vi "CreateNewMissions.vi"(4 "Timeout (s)":dbl, 6 "Duration (s)\n[For in-box mission]":dbl, 8 "Tolerance (m)":dbl, 9 "Mission Type":T3, 10 "Points of Interest":T4[](array[typedef]) {"North" format="%#_10f"; "East" format="%#_8f"}, 11 "Initialized Mission Arrays":T1 {"Readable Missions"."Points of Interest"."North" format="%#_10f"; "Readable Missions"."Points of Interest"."East" format="%#_8f"}) -> (2 "New Mission OUT":refnum<class "GenericMission.lvclass">, 3 "Mission Array Cluster":T1 {"Readable Missions"."Points of Interest"."North" format="%#_10f"; "Readable Missions"."Points of Interest"."East" format="%#_8f"})   [LabVIEW 2013]
doc: "This VI takes in the indicated Mission type and necessary parameters, then creates the Mission object and adds it to\n1) The human readable mission array and\n2) The actual array of mission objects\n\nEric Schneider, August 2014"
uses:
  cRIO_Code/Data/TypeDefs/UTM Location.ctl
  cRIO_Code/Logic/Classes/Missions/GenericMission/GenericMission.lvclass
  cRIO_Code/Data/TypeDefs/MissionTypeControl.ctl
  TypeDef/mission_arrays.ctl
  cRIO_Code/Data/TypeDefs/MissionDescription.ctl
  cRIO_Code/Logic/Classes/Missions/GoTo/GoTo.lvclass
  cRIO_Code/Logic/Classes/Missions/RoundBouy/RoundBouy.lvclass
  cRIO_Code/Logic/Classes/Missions/PassBouy/PassBouy.lvclass
  cRIO_Code/Logic/Classes/Missions/StationKeeping/StationKeeping.lvclass
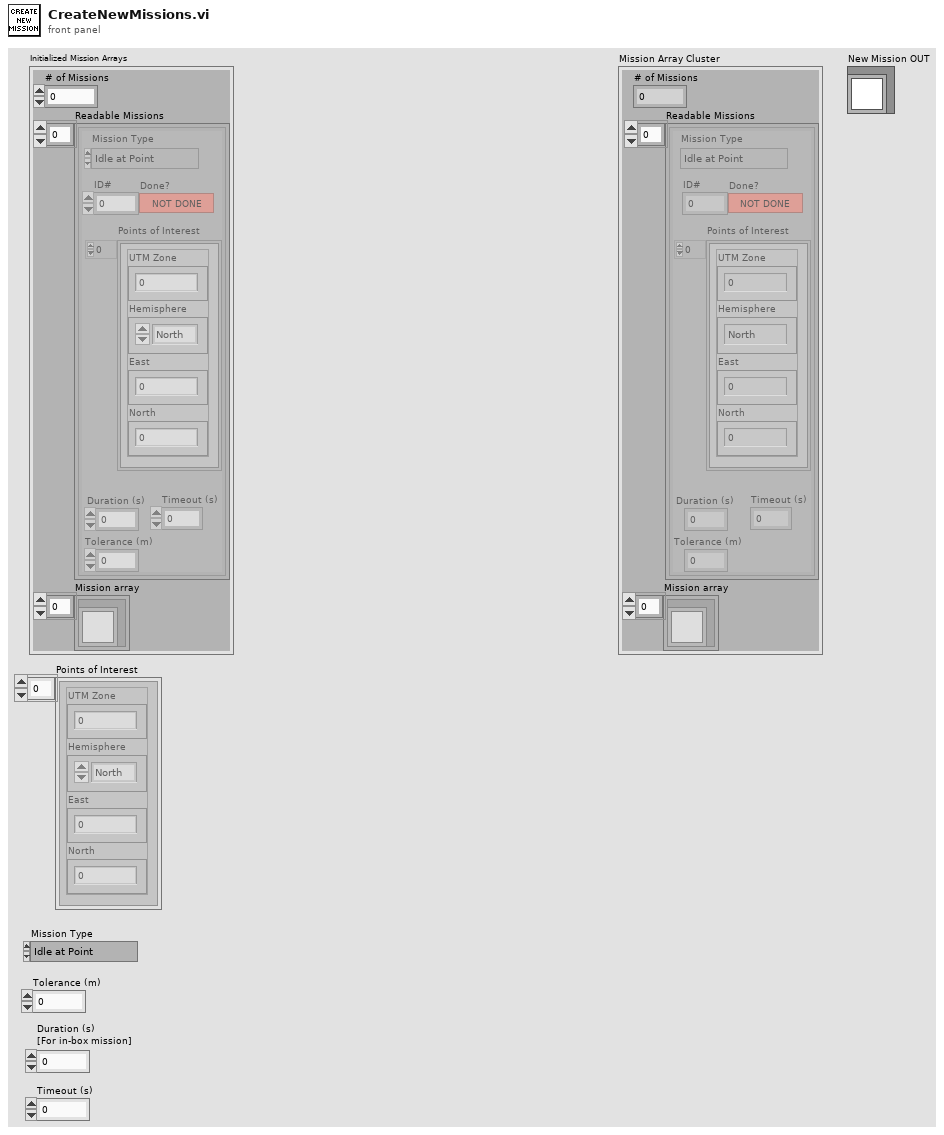
[diagram p1: front panel]
types:
  T1 = typedef "mission_arrays.ctl" = cluster{"# of Missions":i32, "Readable Missions":T2[], "Mission array":refnum<class "GenericMission.lvclass">[]}
  T2 = typedef "MissionDescription.ctl" = cluster{"Duration (s)":dbl, "Timeout (s)":dbl, "Tolerance (m)":dbl, "Mission Type":T3, "Points of Interest":T4[], "ID#":i32, "Done?":bool}
  T3 = typedef "MissionTypeControl.ctl" = enum16{"Idle at Point", "Drive to Waypoint", "Round Buoy to Port", "Round Buoy to Starboard", "Pass Between Buoys", "Station Keeping"}
  T4 = typedef "UTM Location.ctl" = cluster{"UTM Zone":dbl, "Hemisphere":enum16{"North", "South"}, "East":dbl, "North":dbl}
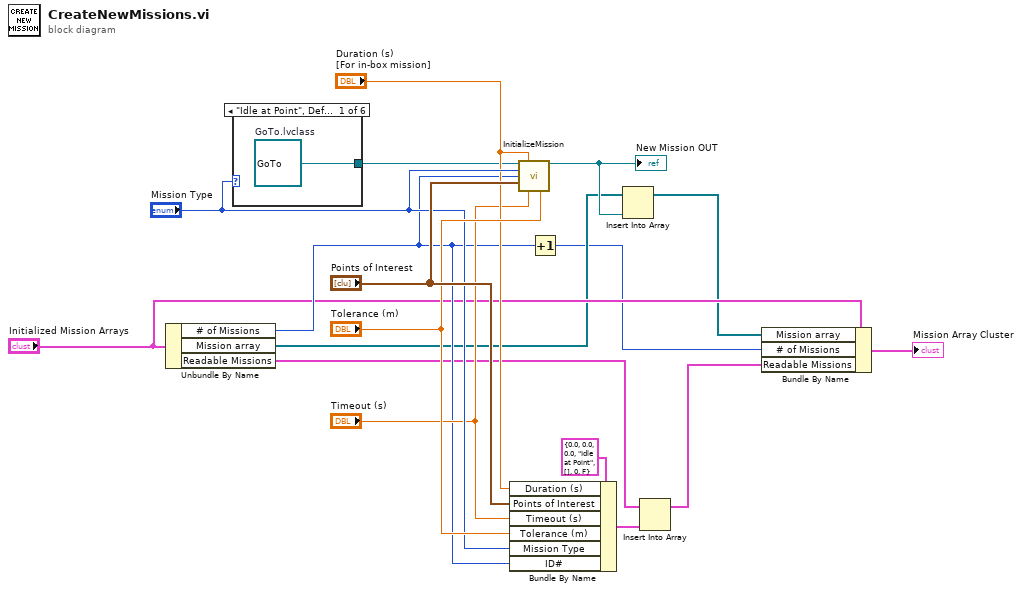
[diagram p0: block diagram]
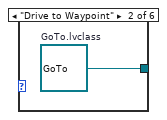
[diagram p2: hidden frame]
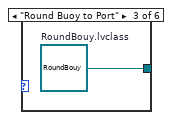
[diagram p3: hidden frame]
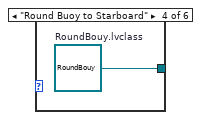
[diagram p4: hidden frame]
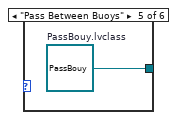
[diagram p5: hidden frame]
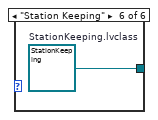
[diagram p6: hidden frame]
diagram:
  n1 = Unbundle By Name("Initialized Mission Arrays") -> ("# of Missions"=w8:i32, "Mission array"=w6:refnum<class "GenericMission.lvclass">[], "Readable Missions"=w5:T2[])
  n2 = case shown="\"Idle at Point\", Default" "Mission Type" {
    tunnel: [w18 w19 w20 w21 w22 w23] -> w9
    frame "Idle at Point", Default {
      w18 = refnum<class "GoTo.lvclass"> refnum  # GoTo.lvclass
    }
    frame "Drive to Waypoint" {
      w19 = refnum<class "GoTo.lvclass"> refnum  # GoTo.lvclass
    }
    frame "Round Buoy to Port" {
      w20 = refnum<class "RoundBouy.lvclass"> refnum  # RoundBouy.lvclass
    }
    frame "Round Buoy to Starboard" {
      w21 = refnum<class "RoundBouy.lvclass"> refnum  # RoundBouy.lvclass
    }
    frame "Pass Between Buoys" {
      w22 = refnum<class "PassBouy.lvclass"> refnum  # PassBouy.lvclass
    }
    frame "Station Keeping" {
      w23 = refnum<class "StationKeeping.lvclass"> refnum  # StationKeeping.lvclass
    }
  }
  n3 = Bundle By Name(cluster=T2 {"Duration (s)"=0.0, "Timeout (s)"=0.0, "Tolerance (m)"=0.0, "Mission Type"=enum."Idle at Point", "Points of Interest"=[], "ID#"=0, "Done?"=FALSE} ("input cluster"), "Duration (s)"="Duration (s)\n[For in-box mission]", "Points of Interest"="Points of Interest", "Timeout (s)"="Timeout (s)", "Tolerance (m)"="Tolerance (m)", "Mission Type"="Mission Type", "ID#"=w8) -> (w11:T2)
  n4 = call-dynamic "InitializeMission.vi"("GenericMission in"=w9, "Duration (s)"="Duration (s)\n[For in-box mission]", "Mission Type"="Mission Type", "ID#"=w8, "Points of Interest"="Points of Interest", "Timeout (s)"="Timeout (s)", "Tolerance (m)"="Tolerance (m)") -> ("GenericMission out"=w16:refnum<class "GenericMission.lvclass">)  [unwired: 7 in, 1 out]
  "New Mission OUT" <- w16
  n5 = Increment(x=w8) -> (x+1=w3:i32)
  n6 = Insert Into Array(array=w6, new element=w16) -> (w2:refnum<class "GenericMission.lvclass">[])  [unwired: 1 in]
  n7 = Insert Into Array(array=w5, new element=w11) -> (w4:T2[])  [unwired: 1 in]
  n8 = Bundle By Name(cluster="Initialized Mission Arrays", "Mission array"=w2, "# of Missions"=w3, "Readable Missions"=w4) -> (→"Mission Array Cluster":T1)
